vi "SRV_JPEGtoPict.vi"(4 "image depth (24)":i32=24, 6 "jpeg string":string, 8 "error in (no error)":errorcluster, 9 "height (240)":i32=240, 10 "width (320)":i32=320, 11 "picture in":picture) -> (0 "error out":errorcluster, 1 "dimensions":cluster{"Width":i32, "Height":i32}, 3 "picture out":picture)   [LabVIEW 2009]
uses:
  <vilib>/picture/picture.llb/imagedata.ctl
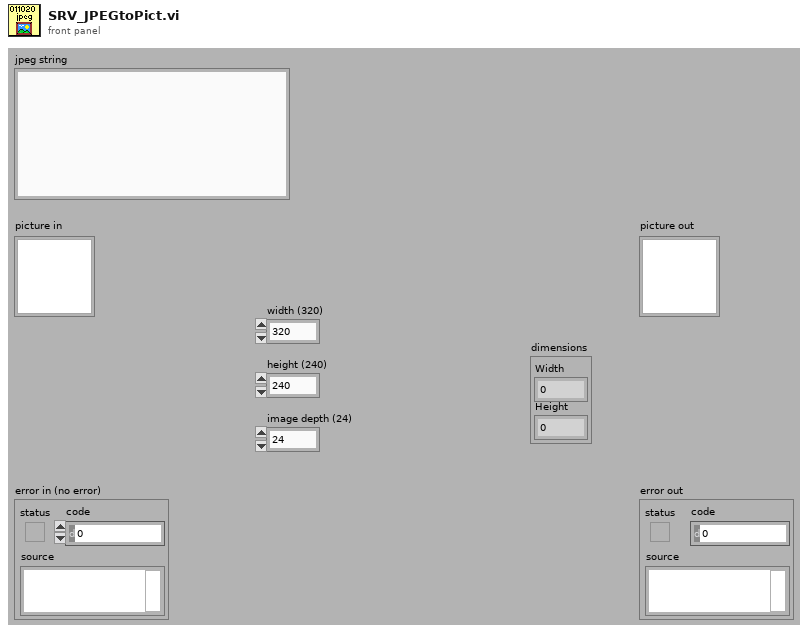
[diagram p1: front panel]
types:
  T1 = typedef "imagedata.ctl" = cluster{"image type":i32, "image depth":i32, "image":u8[], "mask":u8[], "colors":u32[], "Rectangle":cluster{"left":i16, "top":i16, "right":i16, "bottom":i16}}
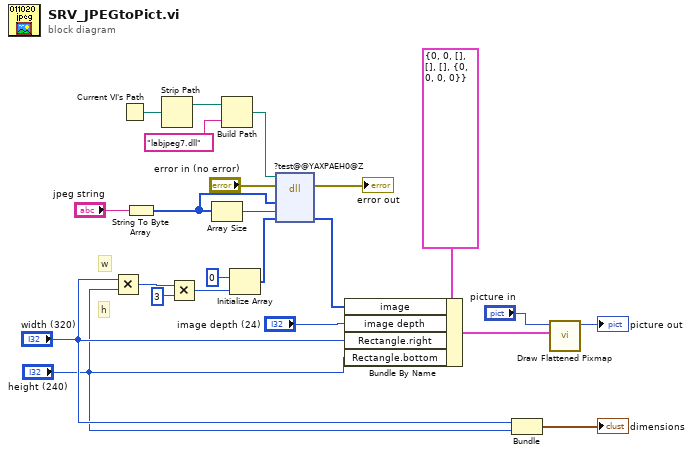
[diagram p0: block diagram]
diagram:
  # "h"
  # "w"
  n1 = Multiply(x="width (320)", y="height (240)") -> (x*y=w22:i32)
  n2 = Current VI's Path() -> (path=w2:path)
  n3 = String To Byte Array(string="jpeg string") -> (unsigned byte array=w10:u8[])
  n4 = Strip Path(path=w2) -> (stripped path=w3:path)  [unwired: 1 out]
  n5 = Multiply(x=w22, y=3) -> (x*y=w20:i32)
  n6 = Array Size(array=w10) -> (size(s)=w23:i32)
  n7 = Build Path(base path=w3, name or relative path="labjpeg7.dll") -> (appended path=w1:path)
  n8 = Initialize Array(u8 0, w20) -> (w18:u8[])
  n9 = dll-call lib="C:/SRV/SRV VIs/ImageProcessing/JPEG to Pict/labjpeg7.dll" fn="?test@@YAXPAEH0@Z"(path in=w1, error in="error in (no error)", "pict"=w10, "size"=w23, "dest"=w18) -> (error out=→"error out":errorcluster, "dest"=w12:u8[])  [unwired: 3 in, 2 out]
  n10 = Bundle By Name(cluster=T1 {"image type"=0, "image depth"=0, "image"=[], "mask"=[], "colors"=[], "Rectangle"={"left"=0, "top"=0, "right"=0, "bottom"=0}} ("image data"), "image"=w12, "image depth"="image depth (24)", "Rectangle.right"="width (320)", "Rectangle.bottom"="height (240)") -> (w14:T1)
  n11 = Bundle("width (320)"="width (320)", "height (240)"="height (240)") -> (→"dimensions":cluster{"width (320)":i32, "height (240)":i32})  [unwired: 1 in]
  n12 = call <vilib>:"Draw Flattened Pixmap.vi"("image data"=w14, "picture"="picture in") -> ("new picture"=→"picture out":picture)  [unwired: 7 out]
